vi "MultiplexerTesting.vi"() -> ()   [LabVIEW 2016]
uses:
  <vilib>/rvi/Emulation/niFpgaGetClockAttributes.vi
  <vilib>/rvi/Emulation/niFpgaSctlEmulationGetInTimedLoop.vi
  <vilib>/rvi/Emulation/niFpgaEmulationReportErrorSimple.vi
  <vilib>/rvi/eio/common/nirviEmuTemplateMethod_errors.vi
  <vilib>/rvi/Emulation/niFpgaCriticalErrorInLSC.vi
  <vilib>/eio/EIONode/EIONode.xnode
panel:
  in  "IN3":u16=1 max=2500 step=25
  in  "IN2":i16=1 min=0 max=550 step=5
  in  "IN1":i16=1 min=0 max=550 step=5
  in  "IN0":u16 max=2500 step=25
  in  "End Program":bool
  in  "INN ->OUT":i8 min=0 max=4 step=1
  # "Voltage Calibration\nThe myRIO attempts to give the following output voltages at these bit values, but doesn't provide enough current at 50 Ohms to achieve it.\n819=1V\n1638=2V\n2457=3V\n\nThese numbers for the voltages sent out from the AO channels  (IN0-IN3 in this vi) are in bits and must be calibrated to your coupling impedance at the OUT of the multiplexer.  Here's what I got in my case.\nVoltage output at 50 Ohms\nIN0 and IN3 MXP (A and B conectors)\n400->0.22V\n800->0.43V\n1200->0.64V\n1600->0.85V\n2000->1.06V\n\nVoltage output at 50 Ohms\nIN1 and IN2 MSP (C connector)\n100->0.21V\n200->0.42V\n300->0.63V\n400->0.84V\n500->1.04V"
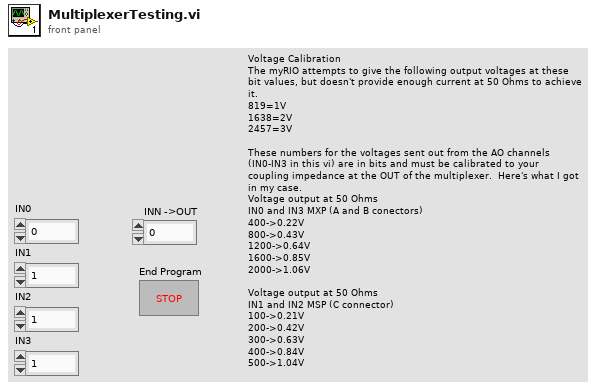
[diagram p1: front panel]
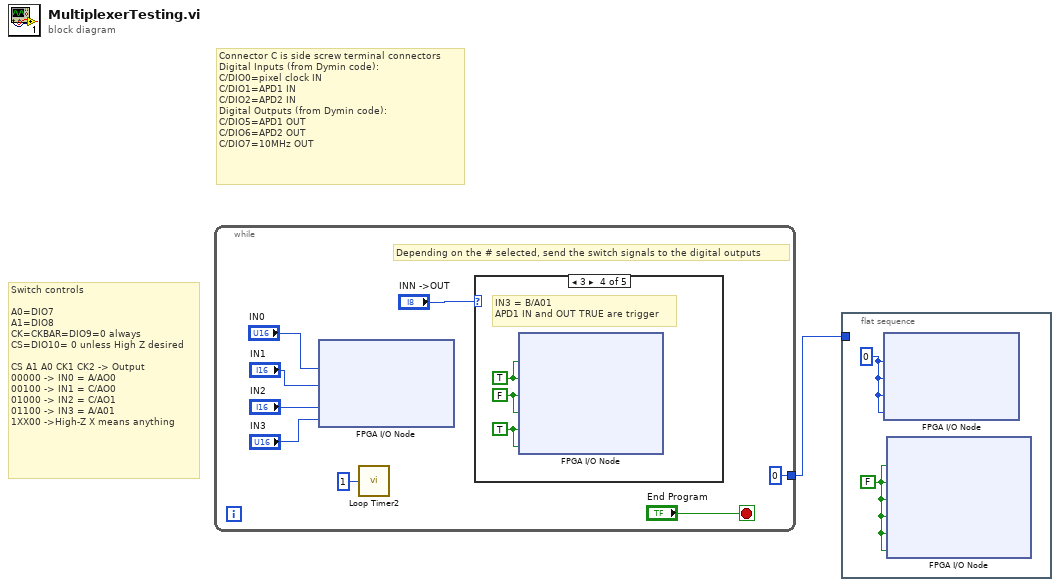
[diagram p0: block diagram]
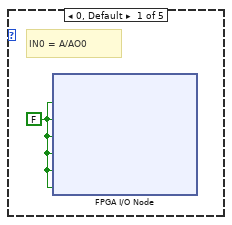
[diagram p2: hidden frame]
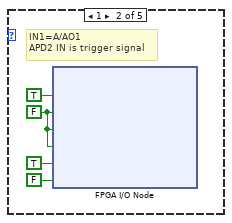
[diagram p3: hidden frame]
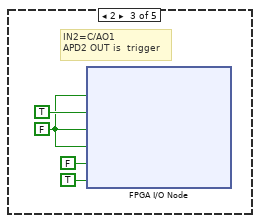
[diagram p4: hidden frame]
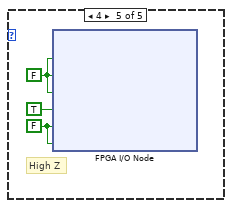
[diagram p5: hidden frame]
diagram:
  # "Switch controls\n\nA0=DIO7\nA1=DIO8\nCK=CKBAR=DIO9=0 always\nCS=DIO10= 0 unless High Z desired\n\nCS A1 A0 CK1 CK2 -> Output\n00000 -> IN0 = A/AO0\n00100 -> IN1 = C/AO0\n01000 -> IN2 = C/AO1\n01100 -> IN3 = A/A01\n1XX00 ->High-Z X means anything"
  # "Connector C is side screw terminal connectors\nDigital Inputs (from Dymin code):\nC/DIO0=pixel clock IN\nC/DIO1=APD1 IN\nC/DIO2=APD2 IN\nDigital Outputs (from Dymin code):\nC/DIO5=APD1 OUT\nC/DIO6=APD2 OUT\nC/DIO7=10MHz OUT"
  n1 = while {
    tunnel: [i8 0 ("switch value of x")] -> w1
    stop <- "End Program" stop-if-true
    # "Depending on the # selected, send the switch signals to the digital outputs"
    n2 = xnode "FPGA I/O Node"("ConnectorA/AO0"="IN0", "ConnectorC/AO0"="IN1", "ConnectorC/AO1"="IN2", "ConnectorA/AO1"="IN3") -> ()  [unwired: 4 in, 4 out]
    n3 = call "Loop Timer2"("Count(Ticks)"=u32 1) -> ()  [unwired: 1 out]
    n4 = case shown="3" "INN ->OUT" {
      frame 0, Default {
        w10 = FALSE ("ConnectorA/DIO0")
        # "IN0 = A/AO0"
        n5 = xnode "FPGA I/O Node"("ConnectorA/DIO7"=w10, "ConnectorA/DIO8"=w10, "ConnectorA/DIO9"=w10, "ConnectorA/DIO10"=w10, "ConnectorC/DIO2"=w10, "ConnectorC/DIO6"=w10) -> ()  [unwired: 6 in, 6 out]
      }
      frame 1 {
        w12 = FALSE ("ConnectorA/DIO1")
        # "IN1=A/AO1\nAPD2 IN is trigger signal"
        n6 = xnode "FPGA I/O Node"("ConnectorA/DIO7"=TRUE, "ConnectorA/DIO8"=w12, "ConnectorA/DIO9"=w12, "ConnectorA/DIO10"=w12, "ConnectorC/DIO2"=TRUE ("ConnectorA/DIO5"), "ConnectorC/DIO6"=FALSE ("ConnectorA/DIO5")) -> ()  [unwired: 6 in, 6 out]
      }
      frame 2 {
        w17 = FALSE
        # "IN2=C/AO1\nAPD2 OUT is  trigger"
        n7 = xnode "FPGA I/O Node"("ConnectorA/DIO7"=w17, "ConnectorA/DIO8"=TRUE ("ConnectorA/DIO3"), "ConnectorA/DIO9"=w17, "ConnectorA/DIO10"=w17, "ConnectorC/DIO2"=FALSE ("ConnectorA/DIO2"), "ConnectorC/DIO6"=TRUE) -> ()  [unwired: 6 in, 6 out]
      }
      frame 3 {
        w19 = TRUE ("ConnectorA/DIO9")
        w20 = FALSE ("ConnectorA/DIO9")
        w21 = TRUE
        # "IN3 = B/A01\nAPD1 IN and OUT TRUE are trigger"
        n8 = xnode "FPGA I/O Node"("ConnectorA/DIO7"=w21, "ConnectorA/DIO8"=w21, "ConnectorA/DIO9"=w20, "ConnectorA/DIO10"=w20, "ConnectorC/DIO2"=w19, "ConnectorC/DIO6"=w19) -> ()  [unwired: 6 in, 6 out]
      }
      frame 4 {
        w22 = FALSE ("ConnectorC/DIO3")
        w24 = FALSE
        # "High Z"
        n9 = xnode "FPGA I/O Node"("ConnectorA/DIO7"=w24, "ConnectorA/DIO8"=w24, "ConnectorA/DIO9"=w24, "ConnectorA/DIO10"=TRUE, "ConnectorC/DIO2"=w22, "ConnectorC/DIO6"=w22) -> ()  [unwired: 6 in, 6 out]
      }
    }
  }
  n10 = flat-sequence {
    tunnel: w1 -> [_]
    frame #0 {
      w26 = u16 0 ("ConnectorA/AO0")
      w25 = FALSE
      n11 = xnode "FPGA I/O Node"("ConnectorA/AO0"=w26, "ConnectorA/AO1"=w26, "ConnectorC/AO0"=w26, "ConnectorC/AO1"=w26) -> ()  [unwired: 4 in, 4 out]
      n12 = xnode "FPGA I/O Node"("ConnectorA/DIO7"=w25, "ConnectorA/DIO8"=w25, "ConnectorA/DIO9"=w25, "ConnectorA/DIO10"=w25, "ConnectorC/DIO2"=w25, "ConnectorC/DIO6"=w25) -> ()  [unwired: 6 in, 6 out]
    }
  }
